vi "HEWH Calculate Valve Position.vi"(8 "Error In":errorcluster, 11 "Core HEWH Data (Input)":T1={"Scan Rate Adjust"=1000.0, "Draw Count"=0, "Test Patten Setup"={"Total Gallons Schedule"=[10.72, 10.72, 10.72, 10.72, 10.72, 10.72], "PRAT/RLT Sequence"=[{"Sequence #"=1.0, "Cycles"=35, "Mode Setting"="", "Flow Rate (GPM)"=0.0, "Temperature (F)"=0.0, "Reset Timer"=FALSE, "Use Temp Decline Method"=FALSE, "Terminate Condition"=enum."C1-Terminate Draw @ Gallon Mark", "Condition Value #1"=0.0, "UE"=FALSE, "LE"=FALSE, "Comp"=FALSE, "Fan"=FALSE, "Test End Time (Sec)"=0.0, "Purge Until Cutout"=FALSE, "Start Conditions"=enum."Heat Source Cutout", "Condition Value #2"=0.0, "Remove Power"=FALSE, "Time"=0.0, "Check Special Cond."=enum."SC1-Do Nothing", "Condition#"=enum."C1", "Draw Flags"=enum."N/A", "Data Processing Delay (FHD 15sec, UEF 5 Sec)"=0.0, "Test Complete"=FALSE}, {"Sequence #"=2.0, "Cycles"=15, "Mode Setting"="", "Flow Rate (GPM)"=0.0, "Temperature (F)"=0.0, "Reset Timer"=FALSE, "Use Temp Decline Method"=FALSE, "Terminate Condition"=enum."C1-Terminate Draw @ Gallon Mark", "Condition Value #1"=0.0, "UE"=FALSE, "LE"=FALSE, "Comp"=FALSE, "Fan"=FALSE, "Test End Time (Sec)"=0.0, "Purge Until Cutout"=FALSE, "Start Conditions"=enum."Heat Source Cutout", "Condition Value #2"=0.0, "Remove Power"=FALSE, "Time"=0.0, "Check Special Cond."=enum."SC1-Do Nothing", "Condition#"=enum."C1", "Draw Flags"=enum."N/A", "Data Processing Delay (FHD 15sec, UEF 5 Sec)"=0.0, "Test Complete"=FALSE}, {"Sequence #"=3.0, "Cycles"=35, "Mode Setting"="", "Flow Rate (GPM)"=0.0, "Temperature (F)"=0.0, "Reset Timer"=FALSE, "Use Temp Decline Method"=FALSE, "Terminate Condition"=enum."C1-Terminate Draw @ Gallon Mark", "Condition Value #1"=0.0, "UE"=FALSE, "LE"=FALSE, "Comp"=FALSE, "Fan"=FALSE, "Test End Time (Sec)"=0.0, "Purge Until Cutout"=FALSE, "Start Conditions"=enum."Heat Source Cutout", "Condition Value #2"=0.0, "Remove Power"=FALSE, "Time"=0.0, "Check Special Cond."=enum."SC1-Do Nothing", "Condition#"=enum."C1", "Draw Flags"=enum."N/A", "Data Processing Delay (FHD 15sec, UEF 5 Sec)"=0.0, "Test Complete"=FALSE}, {"Sequence #"=4.0, "Cycles"=15, "Mode Setting"="", "Flow Rate (GPM)"=0.0, "Temperature (F)"=0.0, "Reset Timer"=FALSE, "Use Temp Decline Method"=FALSE, "Terminate Condition"=enum."C1-Terminate Draw @ Gallon Mark", "Condition Value #1"=0.0, "UE"=FALSE, "LE"=FALSE, "Comp"=FALSE, "Fan"=FALSE, "Test End Time (Sec)"=0.0, "Purge Until Cutout"=FALSE, "Start Conditions"=enum."Heat Source Cutout", "Condition Value #2"=0.0, "Remove Power"=FALSE, "Time"=0.0, "Check Special Cond."=enum."SC1-Do Nothing", "Condition#"=enum."C1", "Draw Flags"=enum."N/A", "Data Processing Delay (FHD 15sec, UEF 5 Sec)"=0.0, "Test Complete"=FALSE}, {"Sequence #"=5.0, "Cycles"=35, "Mode Setting"="", "Flow Rate (GPM)"=0.0, "Temperature (F)"=0.0, "Reset Timer"=FALSE, "Use Temp Decline Method"=FALSE, "Terminate Condition"=enum."C1-Terminate Draw @ Gallon Mark", "Condition Value #1"=0.0, "UE"=FALSE, "LE"=FALSE, "Comp"=FALSE, "Fan"=FALSE, "Test End Time (Sec)"=0.0, "Purge Until Cutout"=FALSE, "Start Conditions"=enum."Heat Source Cutout", "Condition Value #2"=0.0, "Remove Power"=FALSE, "Time"=0.0, "Check Special Cond."=enum."SC1-Do Nothing", "Condition#"=enum."C1", "Draw Flags"=enum."N/A", "Data Processing Delay (FHD 15sec, UEF 5 Sec)"=0.0, "Test Complete"=FALSE}, {"Sequence #"=6.0, "Cycles"=15, "Mode Setting"="", "Flow Rate (GPM)"=0.0, "Temperature (F)"=0.0, "Reset Timer"=FALSE, "Use Temp Decline Method"=FALSE, "Terminate Condition"=enum."C1-Terminate Draw @ Gallon Mark", "Condition Value #1"=0.0, "UE"=FALSE, "LE"=FALSE, "Comp"=FALSE, "Fan"=FALSE, "Test End Time (Sec)"=0.0, "Purge Until Cutout"=FALSE, "Start Conditions"=enum."Heat Source Cutout", "Condition Value #2"=0.0, "Remove Power"=FALSE, "Time"=0.0, "Check Special Cond."=enum."SC1-Do Nothing", "Condition#"=enum."C1", "Draw Flags"=enum."N/A", "Data Processing Delay (FHD 15sec, UEF 5 Sec)"=0.0, "Test Complete"=FALSE}, {"Sequence #"=7.0, "Cycles"=35, "Mode Setting"="", "Flow Rate (GPM)"=0.0, "Temperature (F)"=0.0, "Reset Timer"=FALSE, "Use Temp Decline Method"=FALSE, "Terminate Condition"=enum."C1-Terminate Draw @ Gallon Mark", "Condition Value #1"=0.0, "UE"=FALSE, "LE"=FALSE, "Comp"=FALSE, "Fan"=FALSE, "Test End Time (Sec)"=0.0, "Purge Until Cutout"=FALSE, "Start Conditions"=enum."Heat Source Cutout", "Condition Value #2"=0.0, "Remove Power"=FALSE, "Time"=0.0, "Check Special Cond."=enum."SC1-Do Nothing", "Condition#"=enum."C1", "Draw Flags"=enum."N/A", "Data Processing Delay (FHD 15sec, UEF 5 Sec)"=0.0, "Test Complete"=FALSE}, {"Sequence #"=8.0, "Cycles"=15, "Mode Setting"="", "Flow Rate (GPM)"=0.0, "Temperature (F)"=0.0, "Reset Timer"=FALSE, "Use Temp Decline Method"=FALSE, "Terminate Condition"=enum."C1-Terminate Draw @ Gallon Mark", "Condition Value #1"=0.0, "UE"=FALSE, "LE"=FALSE, "Comp"=FALSE, "Fan"=FALSE, "Test End Time (Sec)"=0.0, "Purge Until Cutout"=FALSE, "Start Conditions"=enum."Heat Source Cutout", "Condition Value #2"=0.0, "Remove Power"=FALSE, "Time"=0.0, "Check Special Cond."=enum."SC1-Do Nothing", "Condition#"=enum."C1", "Draw Flags"=enum."N/A", "Data Processing Delay (FHD 15sec, UEF 5 Sec)"=0.0, "Test Complete"=FALSE}], "Current Sequence Index"=0}, "HEWH Specific DAQ"={"HEWH Data"={"HEWH Standard"={"Voltage (Volts)"=-1.0, "Current (Amps)"=-1.0, "Power (Watts)"=-1.0, "WattHours (Wh)"=-1.0, "TC Tree (AVG)"=0.0, "Flow Rate (GPM)"=0.0, "Gallons (Gal)"=0.0, "RTD Out (Deg F)"=0.0, "RTD In (Deg F)"=0.0, "RTD Amb (Deg F)"=0.0, "TC Down"=0.0, "UE Event Lead"=0, "LE Event Lead"=0, "TC Tree Array"=[]}, "PRAT"={"Power (Watts) A"=4192.0, "Power (Watts) B"=4192.0, "Power (Watts) C"=4192.0, "Power (Watts) D"=4192.0, "TC1"=0.0, "TC2"=0.0, "TC3"=0.0, "TC4"=0.0, "WattHours (Wh) A"=4192.0, "WattHours (Wh) B"=4192.0, "WattHours (Wh) C"=4192.0, "WattHours (Wh) D"=4192.0, "Ambient"=0.0, "Extra Temp"=0.0}, "Additional Power Data"={"Vthd"=236.2, "Frequency (Hz)"=236.2, "Apparent Power (VA)"=236.2, "Power Factor"=236.2, "Current Crest Factor"=236.2, "Voltage Crest Factor"=236.2, "Integration Time (sec)"=236.2}}, "Flow Valve % Open"=0.0, "Power State"={"UE"=FALSE, "LE"=FALSE, "COMP"=FALSE, "FANS"=FALSE}, "Power Analyzer"=enum."APLUS", "Flow Valve uA Output"=0, "Gallons Start (Gal)"=0.0}, "Test Output Data"={"PreDraw Data Table"=[], "Data Table"=[], "MW100 TC Headers"=[]}, "Calc and Calibration"={"Mean SD Var Max Min Array"=[], "Draw Statistics (DBL)"=[], "Calibration Coefficients DBL"=[], "Start Gallons"=0.0, "Starting Temp Decline"=1000.0, "K-Factor (Intellifaucet)"=0.0, "All Draw Stats"=[], "RTD Terminate Value"=0.0}, "Current Draw Time"=0.0, "LV Program"=enum."HEWH", "Station ID"=enum."A", "Current Cond"=enum."N/A", "Test Complete"=FALSE} {"Test Patten Setup"."PRAT/RLT Sequence"."Time" format="%<%H:%M:%S>t"; "Test Patten Setup"."Total Gallons Schedule" format="%.2f"}) -> (0 "Error Out":errorcluster, 2 "Proportional Valve Setting 1":dbl, 3 "Core HEWH Data (Output)":T1={"Scan Rate Adjust"=1000.0, "Draw Count"=0, "Test Patten Setup"={"Total Gallons Schedule"=[10.72, 10.72, 10.72, 10.72, 10.72, 10.72], "PRAT/RLT Sequence"=[{"Sequence #"=1.0, "Cycles"=35, "Mode Setting"="", "Flow Rate (GPM)"=0.0, "Temperature (F)"=0.0, "Reset Timer"=FALSE, "Use Temp Decline Method"=FALSE, "Terminate Condition"=enum."C1-Terminate Draw @ Gallon Mark", "Condition Value #1"=0.0, "UE"=FALSE, "LE"=FALSE, "Comp"=FALSE, "Fan"=FALSE, "Test End Time (Sec)"=0.0, "Purge Until Cutout"=FALSE, "Start Conditions"=enum."Heat Source Cutout", "Condition Value #2"=0.0, "Remove Power"=FALSE, "Time"=0.0, "Check Special Cond."=enum."SC1-Do Nothing", "Condition#"=enum."C1", "Draw Flags"=enum."N/A", "Data Processing Delay (FHD 15sec, UEF 5 Sec)"=0.0, "Test Complete"=FALSE}, {"Sequence #"=2.0, "Cycles"=15, "Mode Setting"="", "Flow Rate (GPM)"=0.0, "Temperature (F)"=0.0, "Reset Timer"=FALSE, "Use Temp Decline Method"=FALSE, "Terminate Condition"=enum."C1-Terminate Draw @ Gallon Mark", "Condition Value #1"=0.0, "UE"=FALSE, "LE"=FALSE, "Comp"=FALSE, "Fan"=FALSE, "Test End Time (Sec)"=0.0, "Purge Until Cutout"=FALSE, "Start Conditions"=enum."Heat Source Cutout", "Condition Value #2"=0.0, "Remove Power"=FALSE, "Time"=0.0, "Check Special Cond."=enum."SC1-Do Nothing", "Condition#"=enum."C1", "Draw Flags"=enum."N/A", "Data Processing Delay (FHD 15sec, UEF 5 Sec)"=0.0, "Test Complete"=FALSE}, {"Sequence #"=3.0, "Cycles"=35, "Mode Setting"="", "Flow Rate (GPM)"=0.0, "Temperature (F)"=0.0, "Reset Timer"=FALSE, "Use Temp Decline Method"=FALSE, "Terminate Condition"=enum."C1-Terminate Draw @ Gallon Mark", "Condition Value #1"=0.0, "UE"=FALSE, "LE"=FALSE, "Comp"=FALSE, "Fan"=FALSE, "Test End Time (Sec)"=0.0, "Purge Until Cutout"=FALSE, "Start Conditions"=enum."Heat Source Cutout", "Condition Value #2"=0.0, "Remove Power"=FALSE, "Time"=0.0, "Check Special Cond."=enum."SC1-Do Nothing", "Condition#"=enum."C1", "Draw Flags"=enum."N/A", "Data Processing Delay (FHD 15sec, UEF 5 Sec)"=0.0, "Test Complete"=FALSE}, {"Sequence #"=4.0, "Cycles"=15, "Mode Setting"="", "Flow Rate (GPM)"=0.0, "Temperature (F)"=0.0, "Reset Timer"=FALSE, "Use Temp Decline Method"=FALSE, "Terminate Condition"=enum."C1-Terminate Draw @ Gallon Mark", "Condition Value #1"=0.0, "UE"=FALSE, "LE"=FALSE, "Comp"=FALSE, "Fan"=FALSE, "Test End Time (Sec)"=0.0, "Purge Until Cutout"=FALSE, "Start Conditions"=enum."Heat Source Cutout", "Condition Value #2"=0.0, "Remove Power"=FALSE, "Time"=0.0, "Check Special Cond."=enum."SC1-Do Nothing", "Condition#"=enum."C1", "Draw Flags"=enum."N/A", "Data Processing Delay (FHD 15sec, UEF 5 Sec)"=0.0, "Test Complete"=FALSE}, {"Sequence #"=5.0, "Cycles"=35, "Mode Setting"="", "Flow Rate (GPM)"=0.0, "Temperature (F)"=0.0, "Reset Timer"=FALSE, "Use Temp Decline Method"=FALSE, "Terminate Condition"=enum."C1-Terminate Draw @ Gallon Mark", "Condition Value #1"=0.0, "UE"=FALSE, "LE"=FALSE, "Comp"=FALSE, "Fan"=FALSE, "Test End Time (Sec)"=0.0, "Purge Until Cutout"=FALSE, "Start Conditions"=enum."Heat Source Cutout", "Condition Value #2"=0.0, "Remove Power"=FALSE, "Time"=0.0, "Check Special Cond."=enum."SC1-Do Nothing", "Condition#"=enum."C1", "Draw Flags"=enum."N/A", "Data Processing Delay (FHD 15sec, UEF 5 Sec)"=0.0, "Test Complete"=FALSE}, {"Sequence #"=6.0, "Cycles"=15, "Mode Setting"="", "Flow Rate (GPM)"=0.0, "Temperature (F)"=0.0, "Reset Timer"=FALSE, "Use Temp Decline Method"=FALSE, "Terminate Condition"=enum."C1-Terminate Draw @ Gallon Mark", "Condition Value #1"=0.0, "UE"=FALSE, "LE"=FALSE, "Comp"=FALSE, "Fan"=FALSE, "Test End Time (Sec)"=0.0, "Purge Until Cutout"=FALSE, "Start Conditions"=enum."Heat Source Cutout", "Condition Value #2"=0.0, "Remove Power"=FALSE, "Time"=0.0, "Check Special Cond."=enum."SC1-Do Nothing", "Condition#"=enum."C1", "Draw Flags"=enum."N/A", "Data Processing Delay (FHD 15sec, UEF 5 Sec)"=0.0, "Test Complete"=FALSE}, {"Sequence #"=7.0, "Cycles"=35, "Mode Setting"="", "Flow Rate (GPM)"=0.0, "Temperature (F)"=0.0, "Reset Timer"=FALSE, "Use Temp Decline Method"=FALSE, "Terminate Condition"=enum."C1-Terminate Draw @ Gallon Mark", "Condition Value #1"=0.0, "UE"=FALSE, "LE"=FALSE, "Comp"=FALSE, "Fan"=FALSE, "Test End Time (Sec)"=0.0, "Purge Until Cutout"=FALSE, "Start Conditions"=enum."Heat Source Cutout", "Condition Value #2"=0.0, "Remove Power"=FALSE, "Time"=0.0, "Check Special Cond."=enum."SC1-Do Nothing", "Condition#"=enum."C1", "Draw Flags"=enum."N/A", "Data Processing Delay (FHD 15sec, UEF 5 Sec)"=0.0, "Test Complete"=FALSE}, {"Sequence #"=8.0, "Cycles"=15, "Mode Setting"="", "Flow Rate (GPM)"=0.0, "Temperature (F)"=0.0, "Reset Timer"=FALSE, "Use Temp Decline Method"=FALSE, "Terminate Condition"=enum."C1-Terminate Draw @ Gallon Mark", "Condition Value #1"=0.0, "UE"=FALSE, "LE"=FALSE, "Comp"=FALSE, "Fan"=FALSE, "Test End Time (Sec)"=0.0, "Purge Until Cutout"=FALSE, "Start Conditions"=enum."Heat Source Cutout", "Condition Value #2"=0.0, "Remove Power"=FALSE, "Time"=0.0, "Check Special Cond."=enum."SC1-Do Nothing", "Condition#"=enum."C1", "Draw Flags"=enum."N/A", "Data Processing Delay (FHD 15sec, UEF 5 Sec)"=0.0, "Test Complete"=FALSE}], "Current Sequence Index"=0}, "HEWH Specific DAQ"={"HEWH Data"={"HEWH Standard"={"Voltage (Volts)"=-1.0, "Current (Amps)"=-1.0, "Power (Watts)"=-1.0, "WattHours (Wh)"=-1.0, "TC Tree (AVG)"=0.0, "Flow Rate (GPM)"=0.0, "Gallons (Gal)"=0.0, "RTD Out (Deg F)"=0.0, "RTD In (Deg F)"=0.0, "RTD Amb (Deg F)"=0.0, "TC Down"=0.0, "UE Event Lead"=0, "LE Event Lead"=0, "TC Tree Array"=[]}, "PRAT"={"Power (Watts) A"=4192.0, "Power (Watts) B"=4192.0, "Power (Watts) C"=4192.0, "Power (Watts) D"=4192.0, "TC1"=0.0, "TC2"=0.0, "TC3"=0.0, "TC4"=0.0, "WattHours (Wh) A"=4192.0, "WattHours (Wh) B"=4192.0, "WattHours (Wh) C"=4192.0, "WattHours (Wh) D"=4192.0, "Ambient"=0.0, "Extra Temp"=0.0}, "Additional Power Data"={"Vthd"=236.2, "Frequency (Hz)"=236.2, "Apparent Power (VA)"=236.2, "Power Factor"=236.2, "Current Crest Factor"=236.2, "Voltage Crest Factor"=236.2, "Integration Time (sec)"=236.2}}, "Flow Valve % Open"=0.0, "Power State"={"UE"=FALSE, "LE"=FALSE, "COMP"=FALSE, "FANS"=FALSE}, "Power Analyzer"=enum."APLUS", "Flow Valve uA Output"=0, "Gallons Start (Gal)"=0.0}, "Test Output Data"={"PreDraw Data Table"=[], "Data Table"=[], "MW100 TC Headers"=[]}, "Calc and Calibration"={"Mean SD Var Max Min Array"=[], "Draw Statistics (DBL)"=[], "Calibration Coefficients DBL"=[], "Start Gallons"=0.0, "Starting Temp Decline"=1000.0, "K-Factor (Intellifaucet)"=0.0, "All Draw Stats"=[], "RTD Terminate Value"=0.0}, "Current Draw Time"=0.0, "LV Program"=enum."HEWH", "Station ID"=enum."A", "Current Cond"=enum."N/A", "Test Complete"=FALSE} {"Test Patten Setup"."PRAT/RLT Sequence"."Time" format="%<%H:%M:%S>t"; "Test Patten Setup"."Total Gallons Schedule" format="%.2f"})   [LabVIEW 2016]
uses:
  Type Definitions/HEWH Output Information.ctl
  Type Definitions/HEWH Draw Pattern Setup.ctl
  Type Definitions/PRAT Test.ctl
  Utility/Save File/File Setup (Public)/Type Definition/Save File HEWH Heating Control Mode.ctl
  Draw Water Specific/Type Definitions/Terminate Draw Conditions.ctl
  Type Definitions/HEWH Start Conditions.ctl
  Draw Water Specific/Type Definitions/Check Special Condtions.ctl
  Draw Water Specific/Type Definitions/HEWH Special Condition Check.ctl
  Type Definitions/HEWH Draw Flag ENUM.ctl
  Type Definitions/HEWH Specific DAQ.ctl
  Type Definitions/HEWH Power Data.ctl
  Type Definitions/HEWH Power Elements.ctl
  Utility/Type Definitions/UTILITY Power Analyzer.ctl
  Type Definitions/HEWH Calc and Calibration.ctl
  Utility/Save File/File Setup (Public)/Type Definition/Save File DOE LabView Program.ctl
  Custom Instrument Control/MW100/Type Definitions/Station ID Selector.ctl
  Utility/Save File/File Setup.lvlib
panel:
  out "Proportional Valve Open Settings":dbl[][](array[numeric])
  # "Draw Pattern Setup (24 Hour)"
  # "Draw Pattern Setup (24 Hour)"
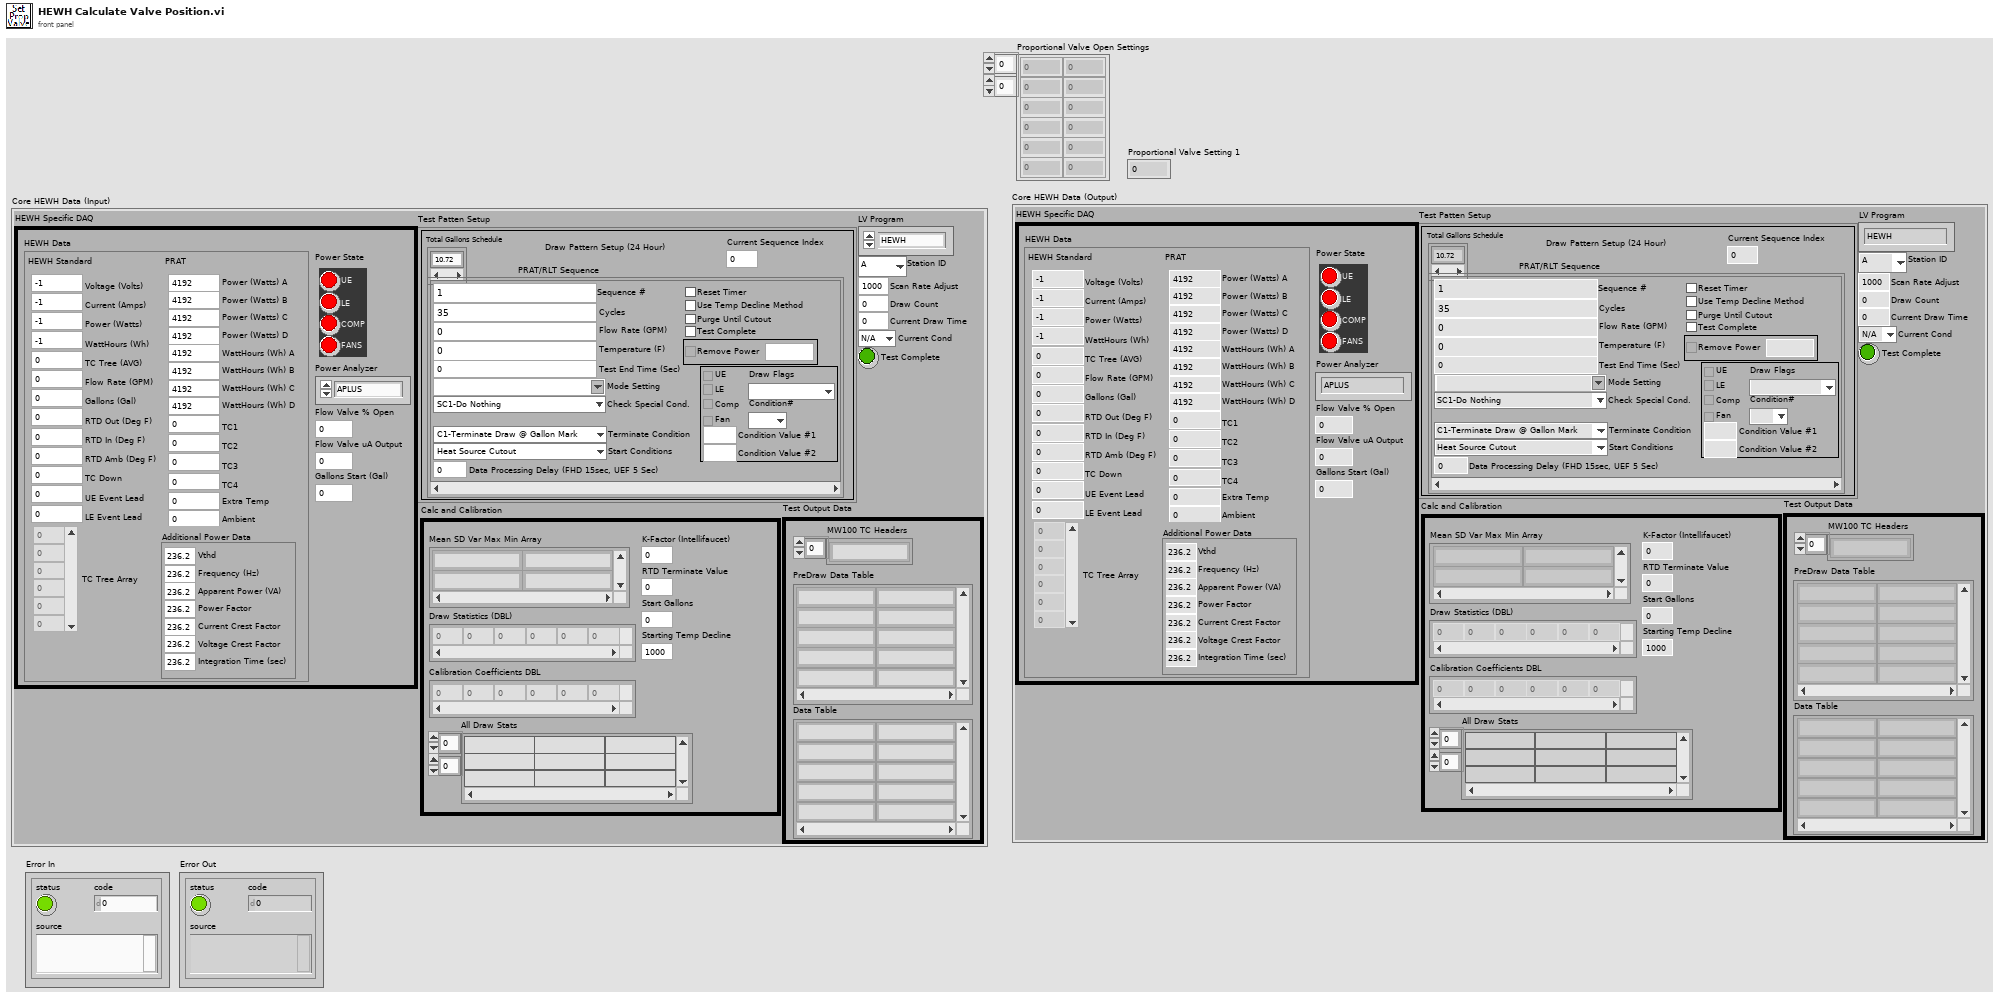
[diagram p1: front panel]
types:
  T1 = typedef "HEWH Output Information.ctl" = cluster{"Scan Rate Adjust":dbl, "Draw Count":i32, "Test Patten Setup":T2, "HEWH Specific DAQ":T10, "Test Output Data":cluster{"PreDraw Data Table":string[][], "Data Table":string[][], "MW100 TC Headers":string[]}, "Calc and Calibration":T14, "Current Draw Time":dbl, "LV Program":T15, "Station ID":T16, "Current Cond":T8, "Test Complete":bool}
  T2 = typedef "HEWH Draw Pattern Setup.ctl" = cluster{"Total Gallons Schedule":dbl[], "PRAT/RLT Sequence":T3[], "Current Sequence Index":i32}
  T3 = typedef "PRAT Test.ctl" = cluster{"Sequence #":dbl, "Cycles":i32, "Mode Setting":T4, "Flow Rate (GPM)":dbl, "Temperature (F)":dbl, "Reset Timer":bool, "Use Temp Decline Method":bool, "Terminate Condition":T5, "Condition Value #1":dbl, "UE":bool, "LE":bool, "Comp":bool, "Fan":bool, "Test End Time (Sec)":dbl, "Purge Until Cutout":bool, "Start Conditions":T6, "Condition Value #2":dbl, "Remove Power":bool, "Time":dbl, "Check Special Cond.":T7, "Condition#":T8, "Draw Flags":T9, "Data Processing Delay (FHD 15sec, UEF 5 Sec)":dbl, "Test Complete":bool}
  T4 = typedef "File Setup.lvlib/Save File HEWH Heating Control Mode.ctl" = string
  T5 = typedef "Terminate Draw Conditions.ctl" = enum16{"C1-Terminate Draw @ Gallon Mark", "C2-Special Last Draw (HU Test)", "C3-RTD Out <=", "C4-Mean Tank Temp <=", "C5-Decrease RTD Out (Deg F)", "C6-Time (Seconds)", "C7-Until Any Heat Source", "C8-Specific Heat Source", "C9-Do Nothing"}
  T6 = typedef "HEWH Start Conditions.ctl" = enum16{"Heat Source Cutout", "At Time (Seconds)", "Every X (Seconds)", "T2 >= X° Below Setpoint", "Seconds From Complete", "Wait for LE & Comp Cutout", "Wait for Comp Cutout", "Wait for LE Cutout", "Wait for UE Cutout"}
  T7 = typedef "Check Special Condtions.ctl" = enum16{"SC1-Do Nothing", "SC2-Check Heat Source (On-C2/Off-C1)", "SC3-Check Skip Condition", "SC4-Check Heat Source ON/Fail"}
  T8 = typedef "HEWH Special Condition Check.ctl" = enum16{"N/A", "C1", "C2", "Reset/Fail", "Skip Draw Sequence"}
  T9 = typedef "HEWH Draw Flag ENUM.ctl" = enum16{"N/A", "None(0)", "Sml(1)", "Med(2)", "SmlMed(3)", "Lrg(4)", "SmlLrg(5)", "MedLrg(6)", "SmlMedLrg(7)"}
  T10 = typedef "HEWH Specific DAQ.ctl" = cluster{"HEWH Data":T11, "Flow Valve % Open":dbl, "Power State":T12, "Power Analyzer":T13, "Flow Valve uA Output":i32, "Gallons Start (Gal)":dbl}
  T11 = typedef "HEWH Power Data.ctl" = cluster{"HEWH Standard":cluster{"Voltage (Volts)":dbl, "Current (Amps)":dbl, "Power (Watts)":dbl, "WattHours (Wh)":dbl, "TC Tree (AVG)":dbl, "Flow Rate (GPM)":dbl, "Gallons (Gal)":dbl, "RTD Out (Deg F)":dbl, "RTD In (Deg F)":dbl, "RTD Amb (Deg F)":dbl, "TC Down":dbl, "UE Event Lead":i32, "LE Event Lead":i32, "TC Tree Array":dbl[]}, "PRAT":cluster{"Power (Watts) A":dbl, "Power (Watts) B":dbl, "Power (Watts) C":dbl, "Power (Watts) D":dbl, "TC1":dbl, "TC2":dbl, "TC3":dbl, "TC4":dbl, "WattHours (Wh) A":dbl, "WattHours (Wh) B":dbl, "WattHours (Wh) C":dbl, "WattHours (Wh) D":dbl, "Ambient":dbl, "Extra Temp":dbl}, "Additional Power Data":cluster{"Vthd":dbl, "Frequency (Hz)":dbl, "Apparent Power (VA)":dbl, "Power Factor":dbl, "Current Crest Factor":dbl, "Voltage Crest Factor":dbl, "Integration Time (sec)":dbl}}
  T12 = typedef "HEWH Power Elements.ctl" = cluster{"UE":bool, "LE":bool, "COMP":bool, "FANS":bool}
  T13 = typedef "UTILITY Power Analyzer.ctl" = enum16{"", "APLUS", "WT210", "WT500", "WT300", "OSI", "Debug", "WT230", "WT300_1", "WT300_2"}
  T14 = typedef "HEWH Calc and Calibration.ctl" = cluster{"Mean SD Var Max Min Array":string[][], "Draw Statistics (DBL)":dbl[][], "Calibration Coefficients DBL":dbl[][], "Start Gallons":dbl, "Starting Temp Decline":dbl, "K-Factor (Intellifaucet)":dbl, "All Draw Stats":string[][], "RTD Terminate Value":dbl}
  T15 = typedef "File Setup.lvlib/Save File DOE LabView Program.ctl" = enum16{"No Name Found", "DOE Stand", "Dishwasher Kitchen", "Portable Stand", "HEWH", "Dryer", "Dryer WILT", "HCC", "PRAT", "HEWH RLT", "Refrigeration"}
  T16 = typedef "Station ID Selector.ctl" = enum16{"", "A", "B", "C", "D", "Global"}
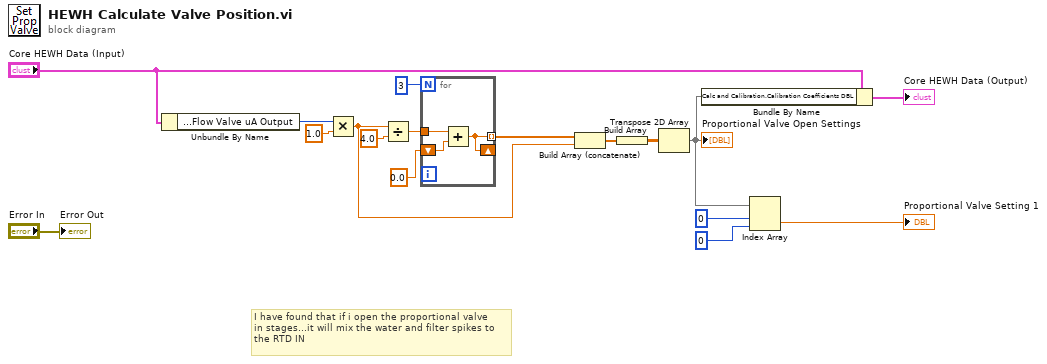
[diagram p0: block diagram]
diagram:
  # "I have found that if i open the proportional valve\nin stages...it will mix the water and filter spikes to\nthe RTD IN"
  n1 = Unbundle By Name("Core HEWH Data (Input)") -> ("HEWH Specific DAQ.Flow Valve uA Output"=w16:i32)
  n2 = Multiply(x=w16, y=1.0) -> (x*y=w10:dbl)
  n3 = Divide(x=w10, y=4.0) -> (x/y=w12:dbl)
  n4 = for {
    N: 3 -> [_]
    tunnel: w12 -> [w20]
    shift-right: [w18] -> _
    shift-left: 0.0 -> [w19]
    tunnel: [w18] -> w1 mode=indexing
    n5 = Add(x=w20, y=w19) -> (x+y=w18:dbl)
  }
  n6 = Build Array (concatenate)(w1, w10) -> (w9:dbl[])
  n7 = Build Array(w9) -> (w7:dbl[][])
  n8 = Transpose 2D Array(2D array=w7) -> (transposed array=w5:dbl[][])
  "Proportional Valve Open Settings" <- w5
  n9 = Bundle By Name(cluster="Core HEWH Data (Input)", "Calc and Calibration.Calibration Coefficients DBL"=w5) -> (→"Core HEWH Data (Output)":T1)
  n10 = Index Array(array=w5, index (row)=0 ("disabled index (row)"), index (col)=0 ("disabled index (col)")) -> (element=→"Proportional Valve Setting 1":dbl)
  "Error Out" <- "Error In"
